vi "Float Value Equal to x Digits.vi"(0 "Value A":ext format="%.16f", 2 "Value B":ext format="%.16f", 6 "Desired Number of matching digits":i32=16) -> (16 "Equal?":bool)   [LabVIEW 2022 SP3, in "Generic Utilities.lvclass"]
doc: "This vi converts a floating point value by first including x decimal number and the converting to a I64. This is needed when performing boolean comparison (is it equal?) of floating value that can be slightly different and one has to be careful when comparing, see <ttp://www.ni.com/white-paper/7612/en/> for more details."
uses:
  Generic Utilities.lvclass
panel:
  out "Number of same digits":i32
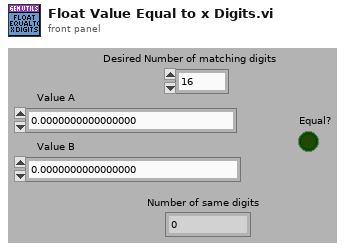
[diagram p1: front panel]
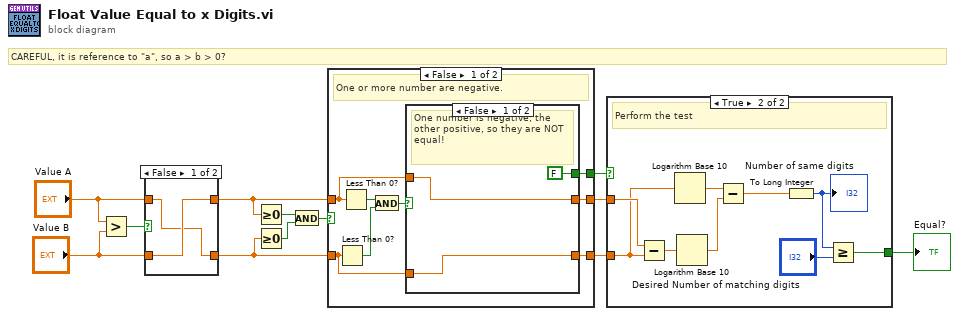
[diagram p0: block diagram]
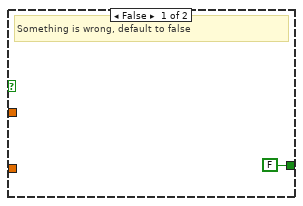
[diagram p2: hidden frame]
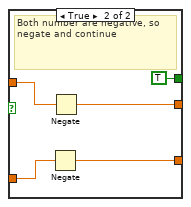
[diagram p3: hidden frame]
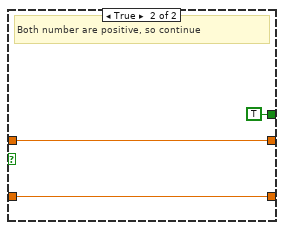
[diagram p4: hidden frame]
diagram:
  # "CAREFUL, it is reference to \"a\", so a > b > 0?"
  n1 = Greater?(x="Value A", y="Value B") -> (0:w11:bool)
  n2 = case shown="False" w11 {
    tunnel: [w14 w16] -> w4
    tunnel: "Value A" -> [w13 w16]
    tunnel: [w13 w15] -> w2
    tunnel: "Value B" -> [w14 w15]
    frame False {
    }
    frame True {
    }
  }
  n3 = Greater Or Equal To 0?(x=w4) -> (x >= 0?=w8:bool)
  n4 = Greater Or Equal To 0?(x=w2) -> (x >= 0?=w7:bool)
  n5 = And(x=w8, y=w7) -> (x .and. y?=w6:bool)
  n6 = case shown="False" w6 {
    tunnel: [w19 w35] -> w5
    tunnel: w4 -> [w20 w35]
    tunnel: [w17 w34] -> w3
    tunnel: w2 -> [w18 w34]
    tunnel: [w21 TRUE] -> w1
    frame False {
      # "One or more number are negative."
      n7 = Less Than 0?(x=w18) -> (x < 0?=w24:bool)
      n8 = Less Than 0?(x=w20) -> (x < 0?=w23:bool)
      n9 = And(x=w23, y=w24) -> (x .and. y?=w22:bool)
      n10 = case shown="False" w22 {
        tunnel: [FALSE TRUE] -> w21
        tunnel: w20 -> [w27 w31]
        tunnel: [w27 w30] -> w19
        tunnel: w18 -> [w26 w29]
        tunnel: [w26 w28] -> w17
        frame False {
          # "One number is negative, the other positive, so they are NOT equal!"
        }
        frame True {
          # "Both number are negative, so negate and continue"
          n11 = Negate(x=w29) -> (-x=w28:ext)
          n12 = Negate(x=w31) -> (-x=w30:ext)
        }
      }
    }
    frame True {
      # "Both number are positive, so continue"
    }
  }
  n13 = case shown="True" w1 {
    tunnel: [FALSE w39] -> w12
    tunnel: w5 -> [_ w38]
    tunnel: w3 -> [_ w37]
    frame False {
      # "Something is wrong, default to false"
    }
    frame True {
      # "Perform the test"
      n14 = Subtract(x=w38, y=w37) -> (x-y=w45:ext)
      n15 = Logarithm Base 10(1:w37) -> (0:w44:ext)
      n16 = Logarithm Base 10(1:w45) -> (0:w43:ext)
      n17 = Subtract(x=w44, y=w43) -> (x-y=w42:ext)
      n18 = To Long Integer(number=w42) -> (32bit integer=w41:i32)
      "Number of same digits" <- w41
      n19 = Greater Or Equal?(x=w41, y="Desired Number of matching digits") -> (x >= y?=w39:bool)
    }
  }
  "Equal?" <- w12
